vi "Send Command.vi"(7 "Data":string, 8 "error in (no error)":errorcluster, 9 "Device and Axis":string, 10 "Command":string, 11 "VISA resource name":refnum<visa-resource-name>) -> (0 "error out":errorcluster, 1 "Response Bundle Array":T2(array[cluster]), 2 "Response String Array":string[](array[string]), 3 "VISA resource name out":refnum<visa-resource-name>, 4 "First Response Bundle":T1, 5 "Number of Replies":i32)   [LabVIEW 2015, in "Zaber A Series.lvlib"]
doc: "Sends a command to the device. For inputting the command, it combines the Device and Axis input, Command input, and Data value input to create a complete command. You could optionally send the complete command directly to the Command input. Omitting the Device and Axis will send the command to all devices/axes. See a command reference here: http://www.zaber.com/wiki/Manuals/ASCII_Protocol_Manual#Command_Reference.\n\nThe Detect Devices VI is designed to provide an easy list of valid Device and Axis inputs. \n\nAn array containing the complete strings of the responses is returned on the Response String Array output, and the details of the format of the response are described here: http://www.zaber.com/wiki/Manuals/ASCII_Protocol_Manual#Replies. This VI also parses the strings, bundles the components, and returns them as an array of bundles on the Response Bundle Array pin. Additionally a pin returns the number of responses received, and a pin returns the First Response Bundle from the Response Bundle Array.\n\nThis VI requires that the Initialize VI has been called with the same serial port."
uses:
  Zaber A Series.lvlib
panel:
  in  "Time per spectrum [ms]":u32=10 max=1000000
  in  "Map points":u32=10
  in  "Acquisition mode":u16(ring) items=["Single spectrum", "Multiple spectra"]
  out "identifier out":string
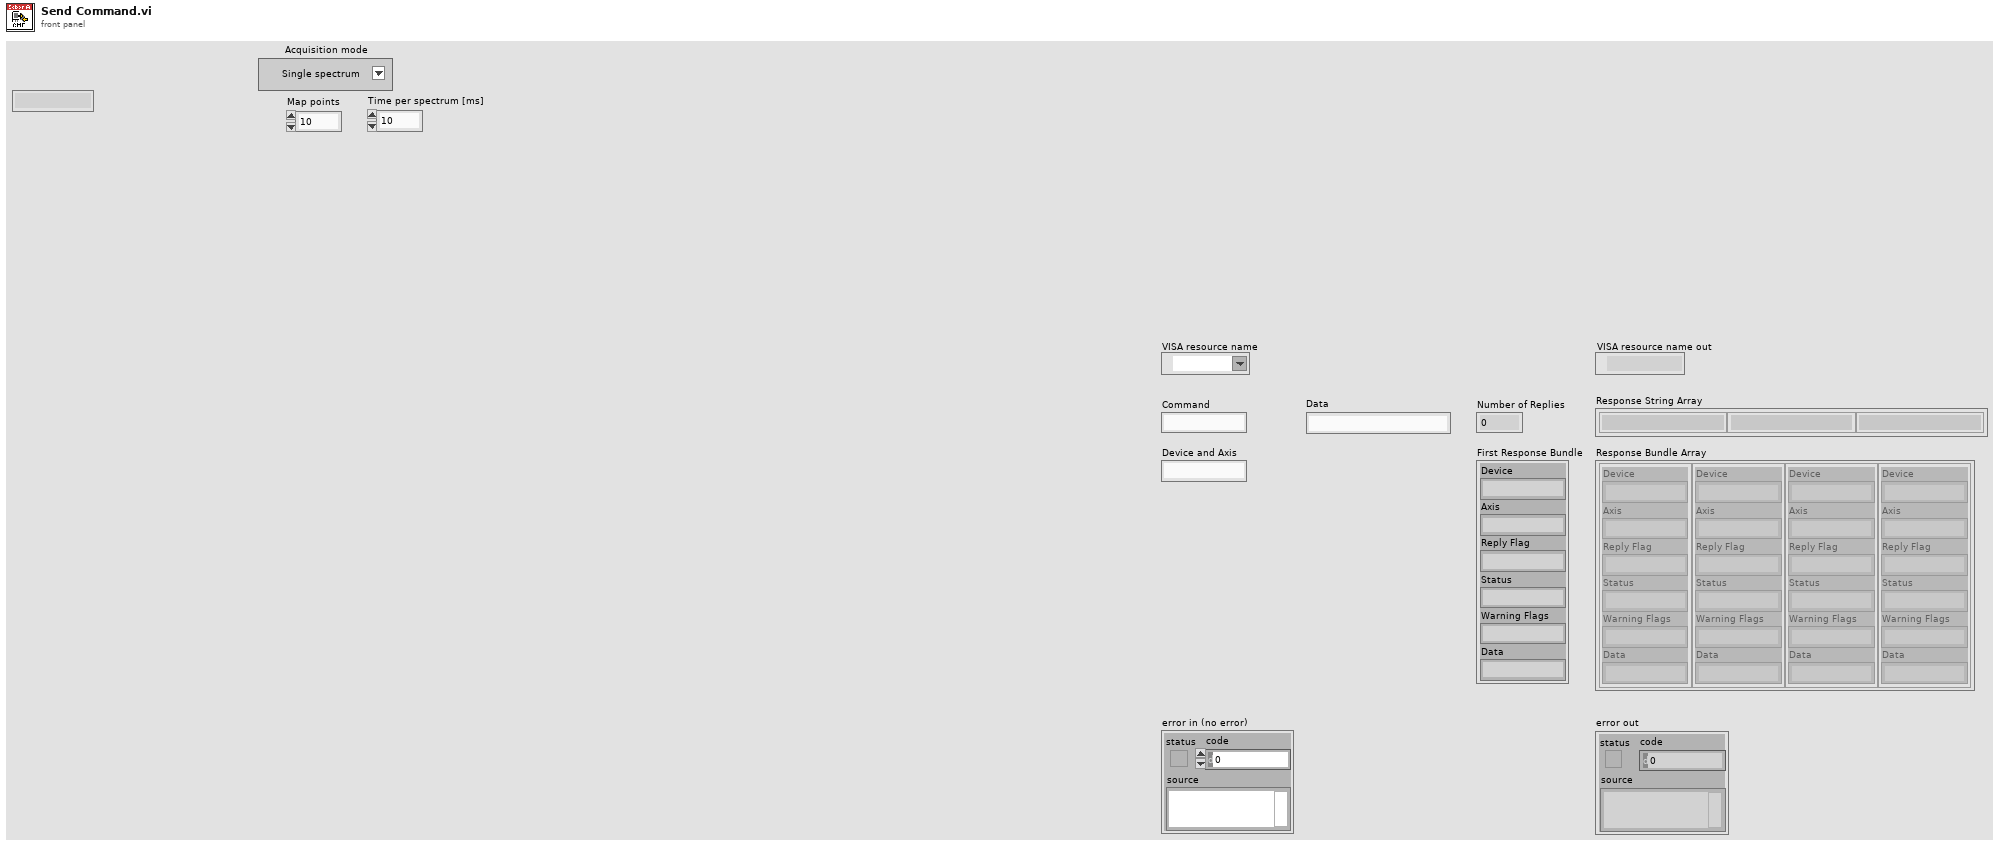
[diagram p1: front panel]
types:
  T1 = cluster{"Device":string, "Axis":string, "Reply Flag":string, "Status":string, "Warning Flags":string, "Data":string}
  T2 = cluster{"Device":string, "Axis":string, "Reply Flag":string, "Status":string, "Warning Flags":string, "Data":string}[]
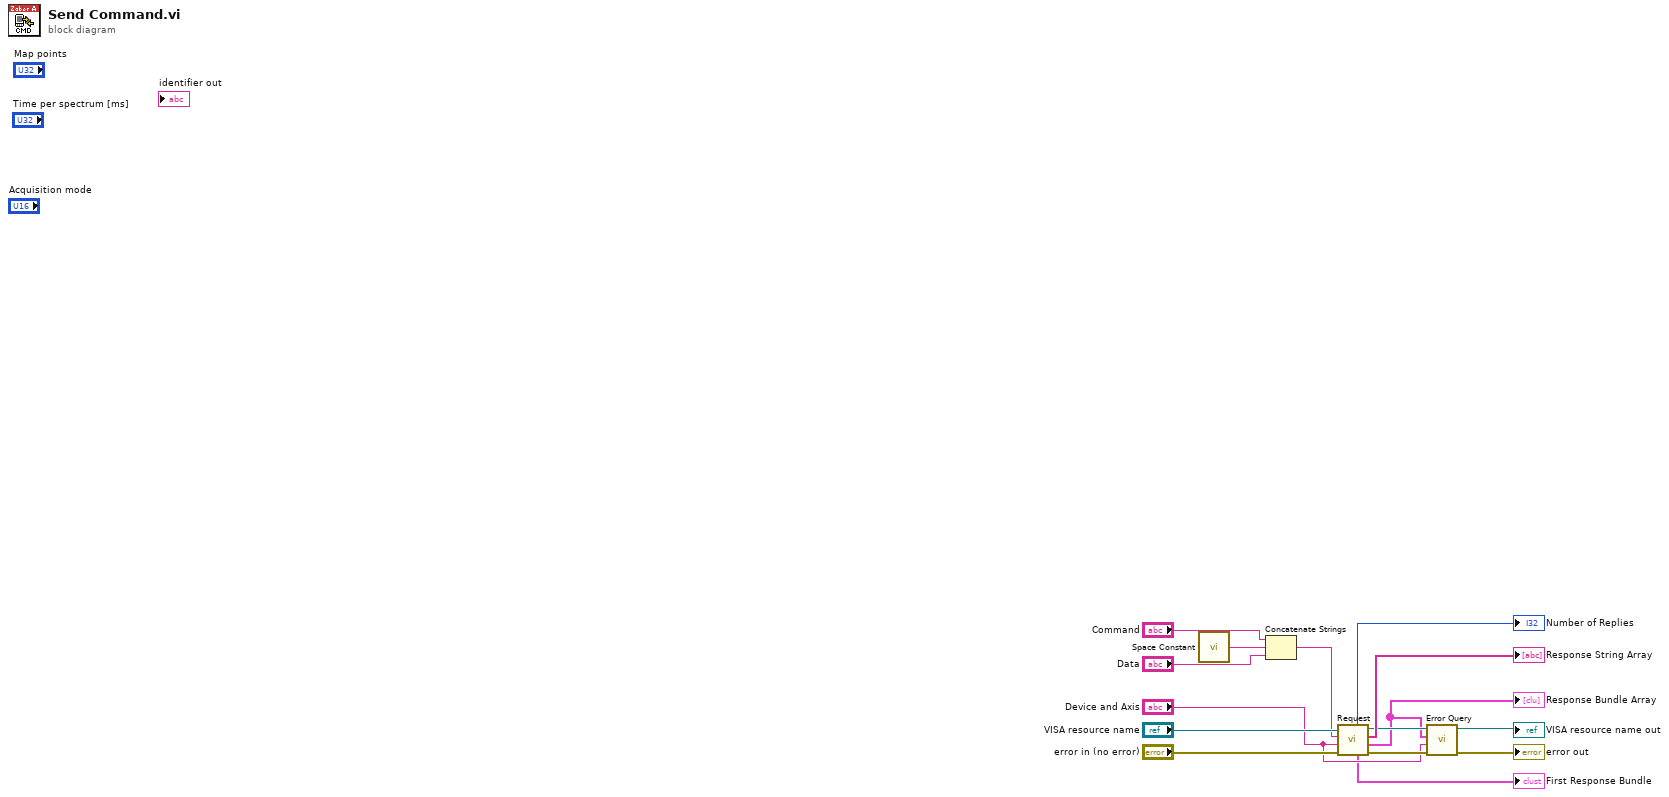
[diagram p0: block diagram]
diagram:
  n1 = call <vilib>:"Space Constant.vi"() -> ("String"=w13:string)
  n2 = Concatenate Strings("Command", w13, "Data") -> (w10:string)
  n3 = call "Request.vi"("error in (no error)"="error in (no error)", "Device and Axis"="Device and Axis", "Command String"=w10, "VISA resource name"="VISA resource name") -> ("error out"=w6:errorcluster, "Response Bundle Array"=w3:T2, "Response String Array"=→"Response String Array":string[], "VISA resource name out"=w7:refnum<visa-resource-name>, "First Response Bundle"=→"First Response Bundle":T1, "Number of Replies"=→"Number of Replies":i32)  [unwired: 2 in]
  "Response Bundle Array" <- w3
  n4 = call "Error Query.vi"("error in (no error)"=w6, "Device and Axis"="Device and Axis", "Previous Response Bundle Array"=w3, "VISA resource name"=w7) -> ("error out"=→"error out":errorcluster, "VISA resource name out"=→"VISA resource name out":refnum<visa-resource-name>)  [unwired: 4 in, 2 out]
